vi "Read Element of Term.vi"(8 "error in (no error)":errorcluster, 10 "index":i32, 11 "State in":refnum<class "State.lvclass">) -> (0 "error out":errorcluster, 2 "Termination":refnum<class "Termination.lvclass">, 3 "State out":refnum<class "State.lvclass">)   [LabVIEW 2020, in "State.lvclass"]
uses:
  State.lvclass
  Termination/Termination.lvclass
  State.lvclass/State.ctl
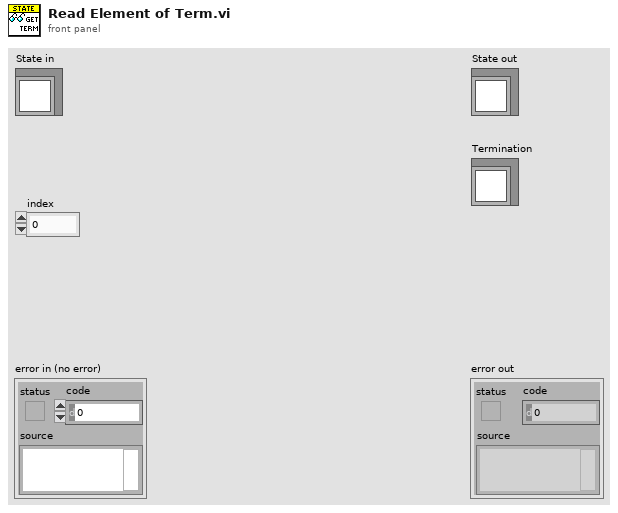
[diagram p1: front panel]
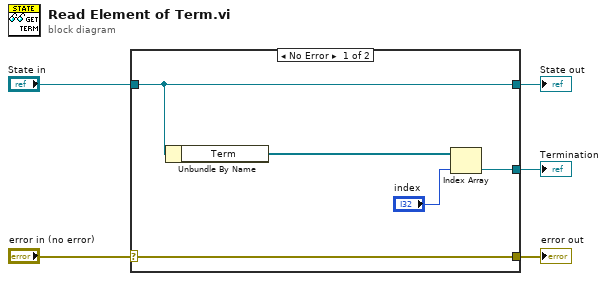
[diagram p0: block diagram]
diagram:
  n1 = case shown="No Error" "error in (no error)" {
    selector: "error in (no error)" -> [w10 w11]
    tunnel: [w10 w11] -> w4
    tunnel: [w9 w12] -> w2
    tunnel: "State in" -> [w9 w12]
    tunnel: [w6 _] -> w1
    frame No Error {
      n2 = Unbundle By Name(w9) -> ("Term"=w8:refnum<class "Termination.lvclass">[])
      n3 = Index Array(array=w8, index="index") -> (element=w6:refnum<class "Termination.lvclass">)
    }
    frame Error {
    }
  }
  "error out" <- w4
  "State out" <- w2
  "Termination" <- w1
